vi "Module-Update.vi"(8 "error in":errorcluster, 11 "UUT":T1) -> (0 "error out":errorcluster)   [LabVIEW 2015, in "Settings-Style.lvlib"]
uses:
  Settings-Style.lvlib
  1_Ctl/DB_UUT.ctl
  1_ctl/Ctl-Color.ctl
  1_Ctl/DB_Update_StateMach.ctl
panel:
  # "Style Settings"
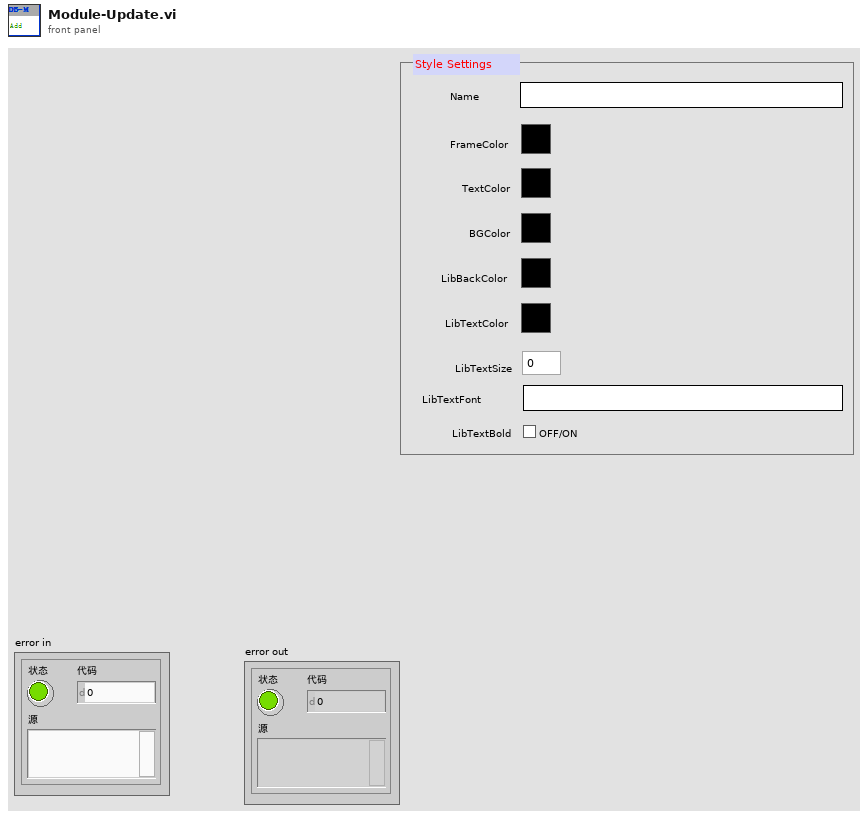
[diagram p1: front panel]
types:
  T1 = typedef "Settings-Style.lvlib/DB_UUT.ctl" = cluster{"Name":string, "FrameColor":T2, "TextColor":T2, "BGColor":T2, "LibBackColor":T2, "LibTextColor":T2, "LibTextSize":u32, "LibTextFont":string, "LibTextBold":bool}
  T2 = typedef "Ctl-Color.ctl" = u32
  T3 = typedef "Settings-Style.lvlib/DB_Update_StateMach.ctl" = enum16{"Initialize", "Update--Begin", "Update-DB_Path_Error", "Update--Check_SN_Exist?", "Update--Done", "Idle", "Error", "WrongState", "Cancel", "SaveData", "Stop"}
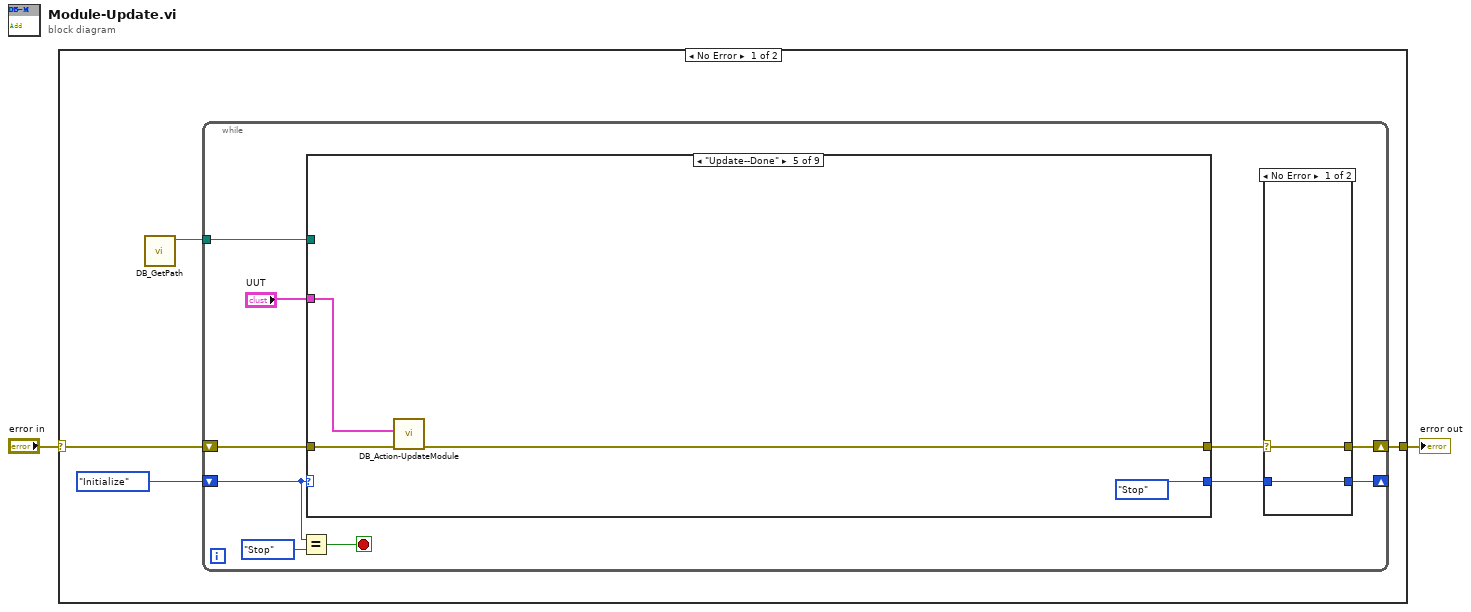
[diagram p0: block diagram]
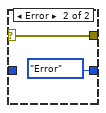
[diagram p2: hidden frame]
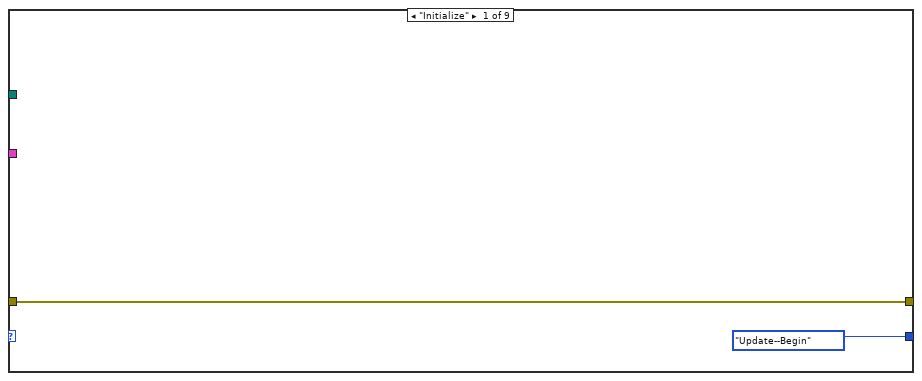
[diagram p3: hidden frame]
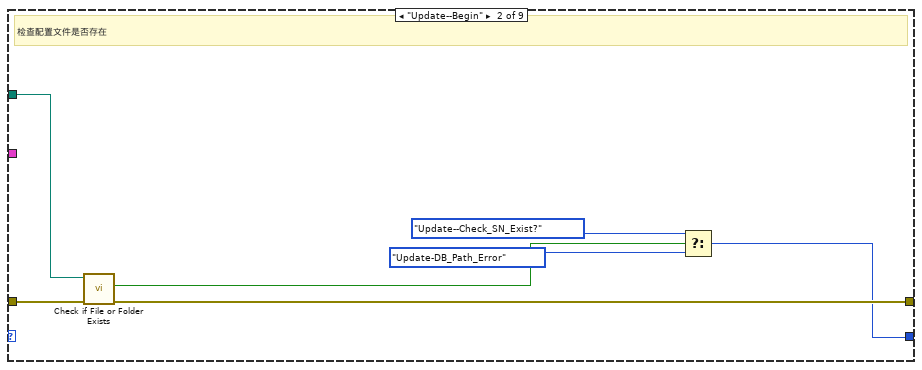
[diagram p4: hidden frame]
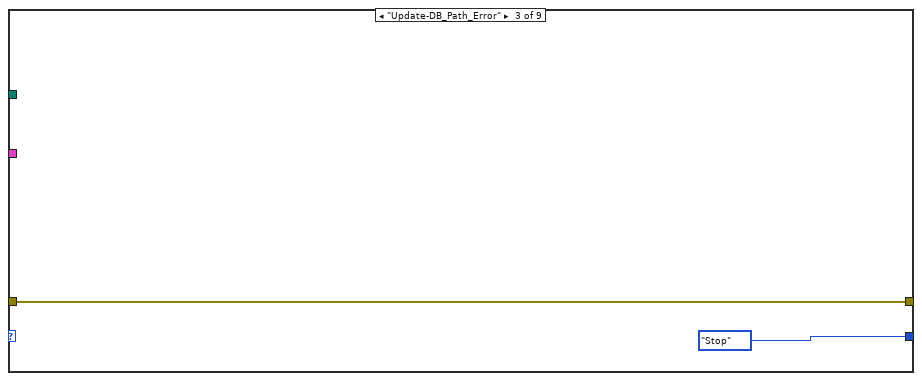
[diagram p5: hidden frame]
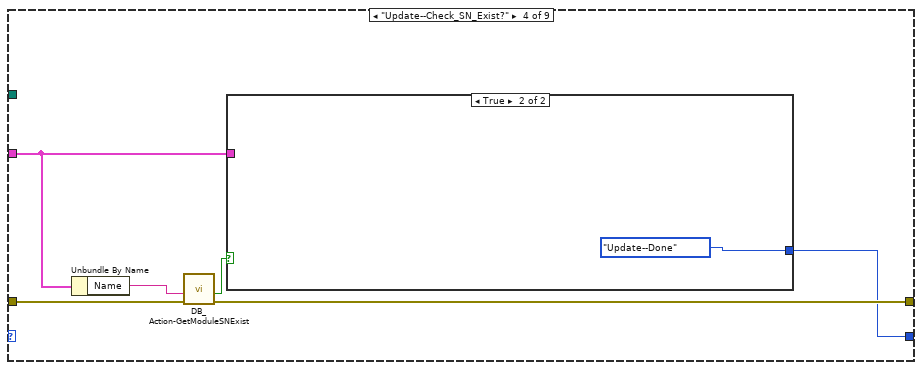
[diagram p6: hidden frame]
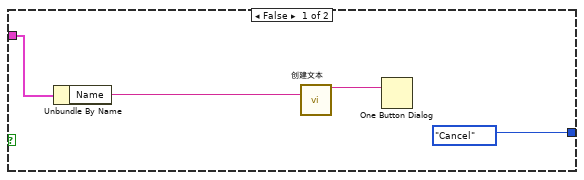
[diagram p7: hidden frame]
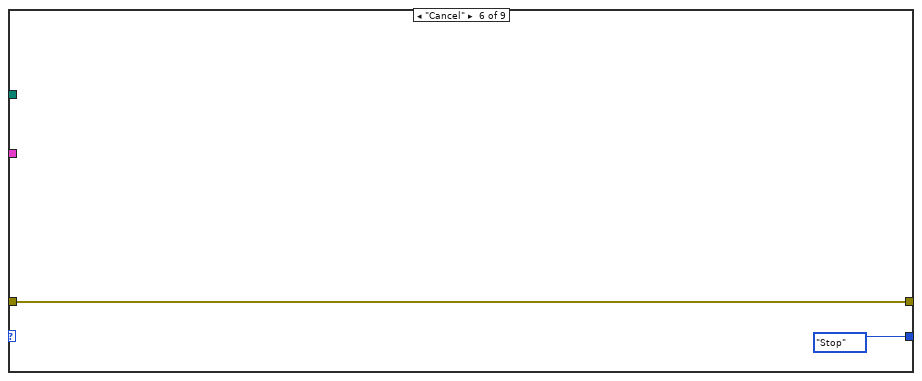
[diagram p8: hidden frame]
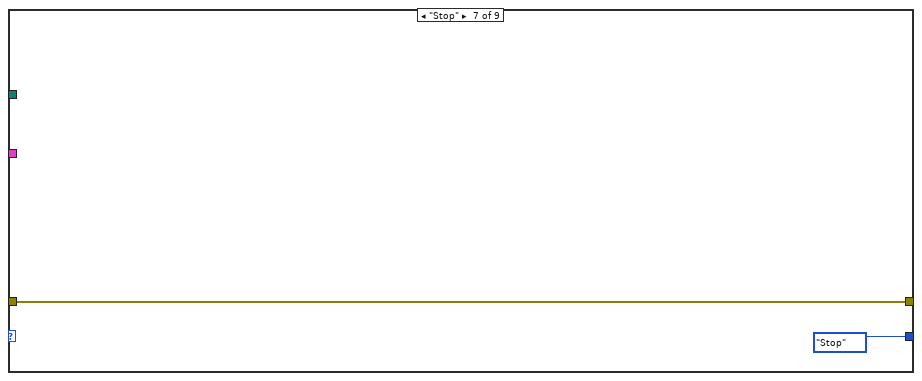
[diagram p9: hidden frame]
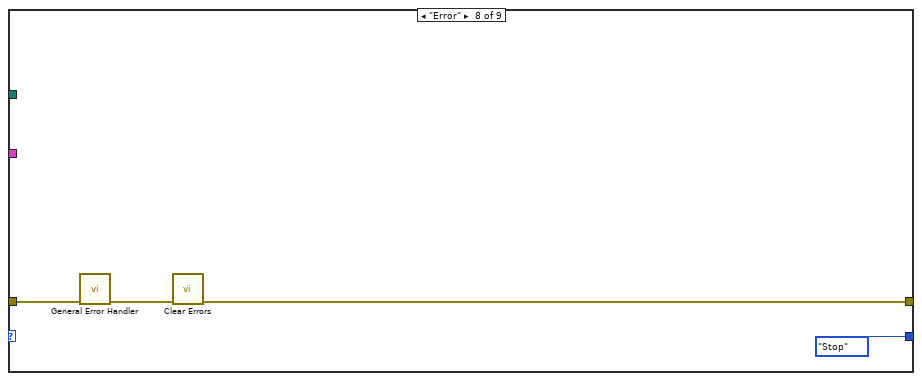
[diagram p10: hidden frame]
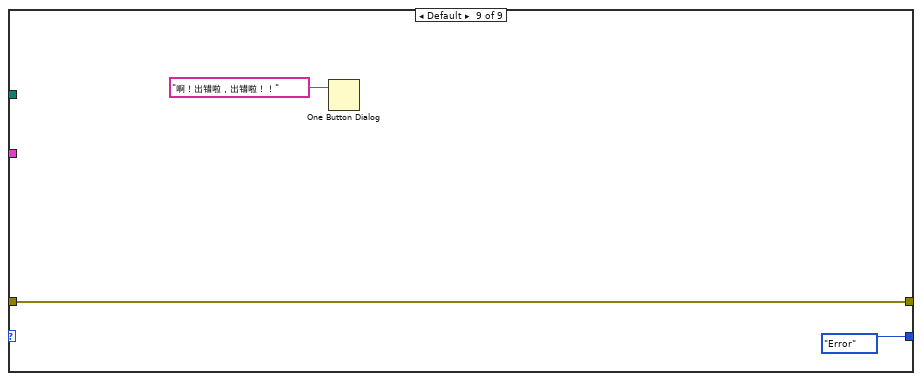
[diagram p11: hidden frame]
diagram:
  n1 = case shown="No Error" "error in" {
    selector: "error in" -> [w5 w58]
    tunnel: [w6 w58] -> w2
    frame No Error {
      n2 = call "DB_GetPath.vi"() -> ("appended path"=w3:path)  [unwired: 11 in]
      n3 = while {
        shift-right: [w10] -> _
        shift-left: DB_Update_StateMach."Initialize" ("Beginning State") -> [w11]
        shift-right: [w12] -> w6
        shift-left: w5 -> [w14]
        tunnel: w3 -> [w8]
        stop <- w16 stop-if-true
        n4 = Equal?(x=w11, y=DB_Update_StateMach."Stop" ("Beginning State")) -> (x = y?=w16:bool)
        n5 = case shown="\"Update--Done\"" w11 {
          tunnel: "UUT" -> [_ _ _ w33 w44 _ _ _ _]
          tunnel: w14 -> [w22 w28 w31 w37 w45 w48 w50 w54 w56]
          tunnel: [w22 w27 w31 w36 w43 w48 w50 w52 w56] -> w13
          tunnel: w8 -> [_ w29 _ _ _ _ _ _ _]
          tunnel: [DB_Update_StateMach."Update--Begin" ("Beginning State") w23 DB_Update_StateMach."Stop" ("Beginning State") w35 DB_Update_StateMach."Stop" ("Beginning State") DB_Update_StateMach."Stop" ("Beginning State") DB_Update_StateMach."Stop" ("Beginning State") DB_Update_StateMach."Stop" ("Beginning State") DB_Update_StateMach."Error" ("Beginning State")] -> w9
          frame "Initialize" {
          }
          frame "Update--Begin" {
            # "检查配置文件是否存在"
            n6 = call <vilib>:"Check if File or Folder Exists.vi"("error in (no error)"=w28, "path"=w29) -> ("error out"=w27:errorcluster, "file or folder exists?"=w26:bool)  [unwired: 7 in, 1 out]
            n7 = Select(t=DB_Update_StateMach."Update--Check_SN_Exist?" ("Beginning State"), s=w26, f=DB_Update_StateMach."Update-DB_Path_Error" ("Beginning State")) -> (s? t:f=w23:T3)
          }
          frame "Update-DB_Path_Error" {
          }
          frame "Update--Check_SN_Exist?" {
            n8 = Unbundle By Name(w33) -> ("Name"=w32:string)
            n9 = call "DB_Action-GetModuleSNExist.vi"("error in"=w37, "Name"=w32) -> ("error out"=w36:errorcluster, "ID_Exist?"=w34:bool)  [unwired: 8 in]
            n10 = case shown="True" w34 {
              tunnel: [DB_Update_StateMach."Cancel" ("Beginning State") DB_Update_StateMach."Update--Done" ("Beginning State")] -> w35
              tunnel: w33 -> [w38 _]
              frame False {
                n11 = Unbundle By Name(w38) -> ("Name"=w39:string)
                n12 = call "创建文本"("Name"=w39) -> ("Result"=w40:string)  [unwired: 13 in, 1 out]
                n13 = One Button Dialog(message=w40) -> ()  [unwired: 1 in, 1 out]
              }
              frame True {
              }
            }
          }
          frame "Update--Done" {
            n14 = call "DB_Action-UpdateModule.vi"("error in"=w45, "UUT输入"=w44) -> ("error out"=w43:errorcluster)  [unwired: 9 in]
          }
          frame "Cancel" {
          }
          frame "Stop" {
          }
          frame "Error" {
            n15 = call <vilib>:"General Error Handler.vi"("error in (no error)"=w54) -> ("error out"=w53:errorcluster)  [unwired: 10 in, 4 out]
            n16 = call <vilib>:"Clear Errors.vi"("error in (no error)"=w53) -> ("error out"=w52:errorcluster)  [unwired: 5 in, 1 out]
          }
          frame Default {
            n17 = One Button Dialog(message="啊！出错啦，出错啦！！" ("消息")) -> ()  [unwired: 1 in, 1 out]
          }
        }
        n18 = case shown="No Error" w13 {
          selector: w13 -> [w18 w20]
          tunnel: [w18 w20] -> w12
          tunnel: [w17 DB_Update_StateMach."Error" ("Beginning State")] -> w10
          tunnel: w9 -> [w17 _]
          frame No Error {
          }
          frame Error {
          }
        }
      }
    }
    frame Error {
    }
  }
  "error out" <- w2
